vi "control final.vi"() -> ()   [LabVIEW 2013]
uses:
  <vilib>/userdefined/High Color/IMAQdx.ctl
  <vilib>/LabVIEW Interface for Arduino/Type Defs/Board Type.ctl
  <vilib>/LabVIEW Interface for Arduino/Type Defs/Connection Type.ctl
  <vilib>/LabVIEW Interface for Arduino/Type Defs/Pin Mode.ctl
  <vilib>/Utility/inputDevices.llb/closeJoystick.vi
  <vilib>/Utility/inputDevices.llb/joystickAcquire.vi
  <vilib>/LabVIEW Interface for Arduino/LabVIEW Interface for Arduino.lvlib
  <vilib>/vision/driver/NI_Vision_Acquisition_Software.lvlib
panel:
  in  "light  2":bool
  in  "light  2":bool
  in  "Session In":T1
  in  "?":bool
  out "CAMERA":T2(plugin-control)
  in  "throtel":dbl(knob) scale=0.0..180.0
  in  "cacamera 2":dbl(knob) scale=0.0..180.0
  in  "laser":bool
  in  "P":bool
  in  "light":bool
  in  "M":bool
  in  "PWM":dbl(knob) scale=0.0..180.0
  out "Voltage":dbl(knob) scale=0.0..5.0
  out "throtel":dbl(knob) scale=0.0..180.0
  out "camera":dbl(knob) scale=0.0..180.0
  out "up":bool
  out "dwn":bool
  out "Rot right":bool
  out "Rot left":bool
  out "gripper":dbl(knob) scale=0.0..180.0
  in  "gripper":dbl(knob) scale=0.0..180.0
  in  "VISA resource":refnum<visa-resource-name>
  out "left":bool
  out "backword":bool
  out "right":bool
  out "forward":bool
  in  "stop":bool
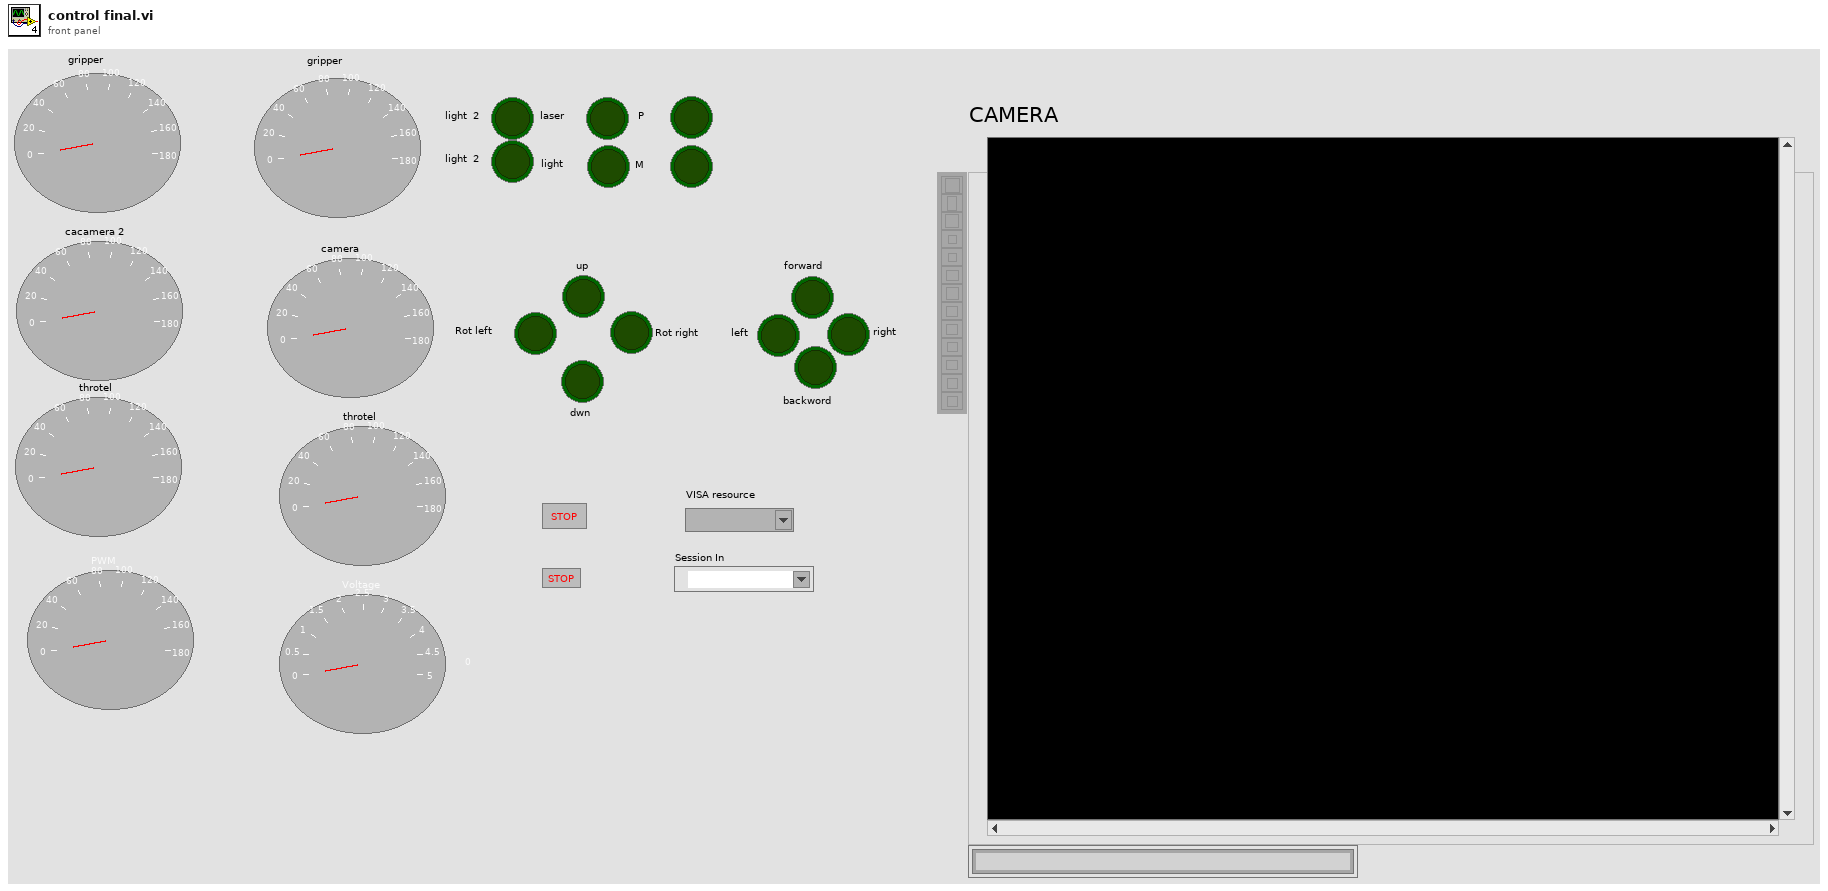
[diagram p1: front panel]
types:
  T1 = typedef "IMAQdx.ctl" = refnum<k21>
  T2 = typedef "IMAQ Image.ctl" = refnum<image>
  T3 = typedef "Image Type" = u32
  T4 = typedef "LabVIEW Interface for Arduino.lvlib/Pin Mode.ctl" = enum8{"Input", "Output"}
  T5 = typedef "LabVIEW Interface for Arduino.lvlib/Connection Type.ctl" = enum8{"USB / Serial", "XBEE", "BlueSmirf (Bluetooth)"}
  T6 = typedef "LabVIEW Interface for Arduino.lvlib/Board Type.ctl" = enum16{"Uno", "Dimuelanove w/Atmega 328", "Mega 2560"}
  T7 = typedef "LabVIEW Interface for Arduino.lvlib/Arduino Resource.ctl" = cluster{"VISA resource":refnum<visa-resource-name>, "Board Type":T6, "Connection Type":enum8{"USB / Serial"}, "Bytes Per Packet (15)":u8}
  T8 = cluster{"X axis":i32, "Y axis":i32, "Z axis":i32, "X axis rotation":i32, "Y axis rotation":i32, "Z axis rotation":i32, "U axis":i32, "V axis":i32}
  T9 = cluster{"button 1":bool, "button 2":bool, "button 3":bool, "button 4":bool, "button 5":bool, "button 6":bool, "button 7":bool, "button 8":bool, "button 9":bool, "button 10":bool, "button 11":bool, "button 12":bool, "button 13":bool, "button 14":bool, "button 15":bool, "button 16":bool, "button 17":bool, "button 18":bool, "button 19":bool, "button 20":bool, "button 21":bool, "button 22":bool, "button 23":bool, "button 24":bool, "button 25":bool, "button 26":bool, "button 27":bool, "button 28":bool, "button 29":bool, "button 30":bool, "button 31":bool, "button 32":bool}
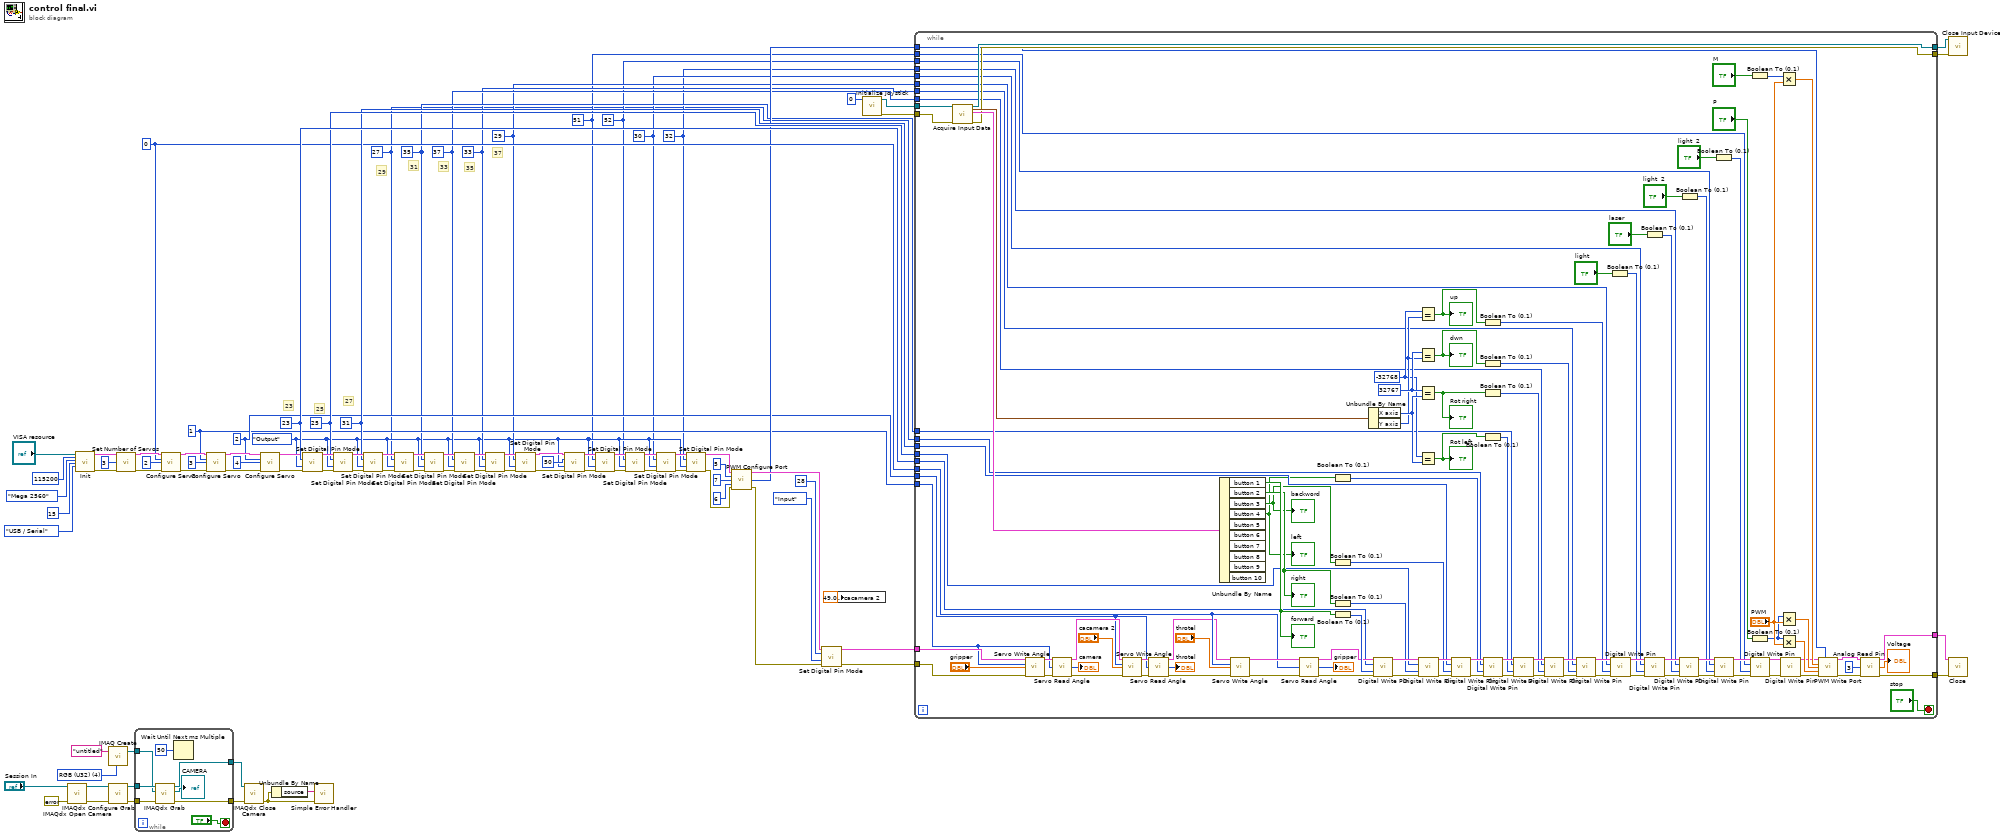
[diagram p0: block diagram]
diagram:
  w8 = T3 4 items=["Grayscale (U8)", "Grayscale (I16)", "Grayscale (SGL)", "Complex (CSG)", "RGB (U32)", "HSL (U32)", "RGB (U64)", "Grayscale (U16)"] ("Image Type")
  w19 = u8 30 ("Digital I/O Pin")
  w18 = u8 32 ("Digital I/O Pin")
  w4 = u8 52 ("Digital I/O Pin")
  w3 = u8 51 ("Digital I/O Pin")
  w24 = u8 29 ("Digital I/O Pin")
  w25 = u8 33 ("Digital I/O Pin")
  w26 = u8 37 ("Digital I/O Pin")
  w27 = u8 35 ("Digital I/O Pin")
  w30 = u8 2 ("Servo Number (0)")
  w29 = u8 1 ("Servo Number (0)")
  w2 = u8 27 ("Value (0)")
  w68 = u8 31 ("Value (0)")
  w69 = u8 25 ("Value (0)")
  w70 = u8 23 ("Value (0)")
  w20 = Pin_Mode."Output" ("Pin Mode (Input)")
  w67 = u8 0 ("Servo Number")
  # "23"
  # "25"
  # "37"
  # "35"
  # "33"
  # "31"
  # "29"
  # "27"
  n1 = call <vilib>:"IMAQdx Open Camera.vi"("error in"=errorcluster {"status"=FALSE, "code"=0, "source"=""}, "Session In"="Session In") -> ("error out"=w12:errorcluster, "Session Out"=w13:T1)  [unwired: 8 in]
  n2 = call <vilib>:"Init.vi"("VISA resource"="VISA resource", "Baud Rate (115200)"=u32 115200, "Board Type (Uno)"=Board_Type."Mega 2560", "Bytes Per Packet (15)"=u32 15, "Connection Type (USB/Serial)"=Connection_Type."USB / Serial") -> ("Arduino Resource"=w78:T7, "error out"=w77:errorcluster)  [unwired: 13 in]
  n3 = call "IMAQ Create"("Image Name"="untitled", "Image Type"=w8) -> ("New Image"=w7:T2)  [unwired: 3 in, 1 out]
  n4 = call <vilib>:"IMAQdx Configure Grab.vi"("error in"=w12, "Session In"=w13) -> ("error out"=w11:errorcluster, "Session Out"=w10:T1)  [unwired: 8 in]
  n5 = call <vilib>:"Set Number of Servos.vi"("Arduino Resource"=w78, "Number Of Servos (1)"=u8 3, "error in"=w77) -> ("Arduino Resource"=w82:T7, "error out"=w81:errorcluster)  [unwired: 11 in]
  n6 = while {
    tunnel: w10 -> [w100]
    tunnel: w11 -> [w99]
    tunnel: [w98] -> w15
    tunnel: [w97] -> w14
    tunnel: w7 -> [w96]
    stop <- "?" stop-if-true
    n7 = call <vilib>:"IMAQdx Grab.vi"("error in"=w99, "Image In"=w96, "Session In"=w100) -> ("error out"=w98:errorcluster, "Image Out"=→"CAMERA":T2, "Session Out"=w97:T1)  [unwired: 5 in, 1 out]
    n8 = Wait Until Next ms Multiple(millisecond multiple=u32 50) -> ()  [unwired: 1 out]
  }
  n9 = call <vilib>:"Configure Servo.vi"("Arduino Resource"=w82, "Servo Number (0)"=w67, "DIO Pin (2)"=u8 2 ("Servo Number"), "error in"=w81) -> ("Arduino Resource"=w51:T7, "error out"=w47:errorcluster)  [unwired: 10 in]
  n10 = call <vilib>:"Configure Servo.vi"("Arduino Resource"=w51, "Servo Number (0)"=w29, "DIO Pin (2)"=u8 3, "error in"=w47) -> ("Arduino Resource"=w50:T7, "error out"=w46:errorcluster)  [unwired: 10 in]
  n11 = call <vilib>:"IMAQdx Close Camera.vi"("error in"=w15, "Session In"=w14) -> ("error out"=w6:errorcluster)  [unwired: 9 in]
  n12 = call <vilib>:"Configure Servo.vi"("Arduino Resource"=w50, "Servo Number (0)"=w30, "DIO Pin (2)"=u8 4, "error in"=w46) -> ("Arduino Resource"=w49:T7, "error out"=w48:errorcluster)  [unwired: 10 in]
  n13 = Unbundle By Name(w6) -> ("source"=w5:string)
  n14 = call <vilib>:"Set Digital Pin Mode.vi"("Arduino Resource"=w49, "Digital I/O Pin"=w70, "Pin Mode (Input)"=w20, "error in"=w48) -> ("Arduino Resource"=w76:T7, "error out"=w71:errorcluster)  [unwired: 10 in]
  n15 = call <vilib>:"Simple Error Handler.vi"("error source (\" \")"=w5, "error in (no error)"=w6) -> ()  [unwired: 3 in, 5 out]
  n16 = call <vilib>:"Set Digital Pin Mode.vi"("Arduino Resource"=w76, "Digital I/O Pin"=w69, "Pin Mode (Input)"=w20, "error in"=w71) -> ("Arduino Resource"=w75:T7, "error out"=w72:errorcluster)  [unwired: 10 in]
  n17 = call <vilib>:"Set Digital Pin Mode.vi"("Arduino Resource"=w75, "Digital I/O Pin"=w68, "Pin Mode (Input)"=w20, "error in"=w72) -> ("Arduino Resource"=w74:T7, "error out"=w73:errorcluster)  [unwired: 10 in]
  n18 = call <vilib>:"Set Digital Pin Mode.vi"("Arduino Resource"=w74, "Digital I/O Pin"=w2, "Pin Mode (Input)"=w20, "error in"=w73) -> ("Arduino Resource"=w65:T7, "error out"=w52:errorcluster)  [unwired: 10 in]
  n19 = call <vilib>:"Set Digital Pin Mode.vi"("Arduino Resource"=w65, "Digital I/O Pin"=w27, "Pin Mode (Input)"=w20, "error in"=w52) -> ("Arduino Resource"=w64:T7, "error out"=w53:errorcluster)  [unwired: 10 in]
  n20 = call <vilib>:"Set Digital Pin Mode.vi"("Arduino Resource"=w64, "Digital I/O Pin"=w26, "Pin Mode (Input)"=w20, "error in"=w53) -> ("Arduino Resource"=w63:T7, "error out"=w54:errorcluster)  [unwired: 10 in]
  n21 = call <vilib>:"Set Digital Pin Mode.vi"("Arduino Resource"=w63, "Digital I/O Pin"=w25, "Pin Mode (Input)"=w20, "error in"=w54) -> ("Arduino Resource"=w62:T7, "error out"=w55:errorcluster)  [unwired: 10 in]
  n22 = call <vilib>:"Set Digital Pin Mode.vi"("Arduino Resource"=w62, "Digital I/O Pin"=w24, "Pin Mode (Input)"=w20, "error in"=w55) -> ("Arduino Resource"=w61:T7, "error out"=w56:errorcluster)  [unwired: 10 in]
  n23 = call <vilib>:"Set Digital Pin Mode.vi"("Arduino Resource"=w61, "Digital I/O Pin"=u8 50, "Pin Mode (Input)"=w20, "error in"=w56) -> ("Arduino Resource"=w60:T7, "error out"=w57:errorcluster)  [unwired: 10 in]
  n24 = call <vilib>:"Set Digital Pin Mode.vi"("Arduino Resource"=w60, "Digital I/O Pin"=w3, "Pin Mode (Input)"=w20, "error in"=w57) -> ("Arduino Resource"=w59:T7, "error out"=w58:errorcluster)  [unwired: 10 in]
  n25 = call <vilib>:"Set Digital Pin Mode.vi"("Arduino Resource"=w59, "Digital I/O Pin"=w4, "Pin Mode (Input)"=w20, "error in"=w58) -> ("Arduino Resource"=w22:T7, "error out"=w21:errorcluster)  [unwired: 10 in]
  n26 = call <vilib>:"Set Digital Pin Mode.vi"("Arduino Resource"=w22, "Digital I/O Pin"=w19, "Pin Mode (Input)"=w20, "error in"=w21) -> ("Arduino Resource"=w40:T7, "error out"=w39:errorcluster)  [unwired: 10 in]
  n27 = call <vilib>:"Set Digital Pin Mode.vi"("Arduino Resource"=w40, "Digital I/O Pin"=w18, "Pin Mode (Input)"=w20, "error in"=w39) -> ("Arduino Resource"=w38:T7, "error out"=w37:errorcluster)  [unwired: 10 in]
  n28 = call <vilib>:"PWM Configure Port.vi"("Arduino Resource"=w38, "PWM Pin (3)"=u8 5, "PWM Pin (5)"=u8 7, "PWM Pin (6)"=u8 6, "error in"=w37) -> ("Arduino Resource"=w35:T7, "PWM Pins"=w31:u8[], "error out"=w36:errorcluster)  [unwired: 8 in]
  n29 = call <vilib>:"Set Digital Pin Mode.vi"("Arduino Resource"=w35, "Digital I/O Pin"=u8 28, "Pin Mode (Input)"=Pin_Mode."Input", "error in"=w36) -> ("Arduino Resource"=w42:T7, "error out"=w43:errorcluster)  [unwired: 10 in]
  n30 = local write "cacamera 2"(49.0 ("caca 2")) -> ()
  n31 = call <vilib>:"Initialize Joystick.vi"("device index"=0) -> ("error out"=w88:errorcluster, "device ID"=w89:refnum<k1>)  [unwired: 9 in]
  n32 = while {
    tunnel: w89 -> [w211]
    tunnel: w88 -> [w210]
    tunnel: [w167] -> w87
    tunnel: [w166] -> w86
    tunnel: [w203] -> w85
    tunnel: [w202] -> w84
    tunnel: w70 -> [w175]
    tunnel: w69 -> [w174]
    tunnel: w68 -> [w173]
    tunnel: w2 -> [w172]
    tunnel: w67 -> [w171]
    tunnel: w42 -> [w144]
    tunnel: w43 -> [w143]
    tunnel: w31 -> [w154]
    tunnel: w30 -> [w139]
    tunnel: w29 -> [w140]
    tunnel: w27 -> [w138]
    tunnel: w26 -> [w137]
    tunnel: w25 -> [w136]
    tunnel: w24 -> [w135]
    tunnel: w19 -> [w120]
    tunnel: w18 -> [w119]
    tunnel: w4 -> [w104]
    tunnel: w3 -> [w103]
    stop <- "stop" stop-if-true
    w204 = -32768 ("x")
    w206 = 32767 ("x")
    n33 = call-poly <vilib>:"Acquire Input Data.vi"("device ID"=w211, "error in (no error)"=w210) -> ("device ID"=w203:refnum<k1>, "axis info"=w208:T8, "button info"=w209:T9, "error out"=w202:errorcluster)  [unwired: 13 in, 1 out]
    n34 = call <vilib>:"Servo Write Angle.vi"("Arduino Resource"=w144, "Servo Number"=w140, "Angle (Degrees)"="gripper", "error in"=w143) -> ("Arduino Resource"=w149:T7, "error out"=w152:errorcluster)  [unwired: 10 in]
    n35 = call <vilib>:"Servo Read Angle.vi"("Arduino Resource"=w149, "Servo Number"=w140, "error in"=w152) -> ("Arduino Resource"=w150:T7, "Angle (Degrees)"=→"camera":u8, "error out"=w148:errorcluster)  [unwired: 10 in]
    n36 = call <vilib>:"Servo Write Angle.vi"("Arduino Resource"=w150, "Servo Number"=w139, "Angle (Degrees)"="cacamera 2", "error in"=w148) -> ("Arduino Resource"=w151:T7, "error out"=w153:errorcluster)  [unwired: 10 in]
    n37 = call <vilib>:"Servo Read Angle.vi"("Arduino Resource"=w151, "Servo Number"=w139, "error in"=w153) -> ("Arduino Resource"=w146:T7, "Angle (Degrees)"=→"throtel":u8, "error out"=w147:errorcluster)  [unwired: 10 in]
    n38 = Unbundle By Name(w209) -> ("button 1"=w201:bool, "button 2"=w200:bool, "button 3"=w199:bool, "button 4"=w129:bool)  [unwired: 6 out]
    "forward" <- w201
    "right" <- w200
    "backword" <- w199
    "left" <- w129
    n39 = call <vilib>:"Servo Write Angle.vi"("Arduino Resource"=w146, "Servo Number"=w171, "Angle (Degrees)"="throtel", "error in"=w147) -> ("Arduino Resource"=w179:T7, "error out"=w178:errorcluster)  [unwired: 10 in]
    n40 = call <vilib>:"Servo Read Angle.vi"("Arduino Resource"=w179, "Servo Number"=w171, "error in"=w178) -> ("Arduino Resource"=w177:T7, "Angle (Degrees)"=→"gripper":u8, "error out"=w176:errorcluster)  [unwired: 10 in]
    n41 = Boolean To (0,1)(Boolean=w129) -> (0, 1=w184:i16)
    n42 = Boolean To (0,1)(Boolean=w199) -> (0, 1=w183:i16)
    n43 = Boolean To (0,1)(Boolean=w200) -> (0, 1=w182:i16)
    n44 = Boolean To (0,1)(Boolean=w201) -> (0, 1=w181:i16)
    n45 = Unbundle By Name(w208) -> ("X axis"=w207:i32, "Y axis"=w205:i32)
    n46 = call <vilib>:"Digital Write Pin.vi"("Arduino Resource"=w177, "Digital I/O Pin (0)"=w175, "Value (0)"=w181, "error in"=w176) -> ("Arduino Resource"=w193:T7, "error out"=w196:errorcluster)  [unwired: 10 in]
    n47 = Equal?(x=w204, y=w205) -> (x = y?=w160:bool)
    "up" <- w160
    n48 = Equal?(x=w206, y=w205) -> (x = y?=w161:bool)
    "dwn" <- w161
    n49 = Equal?(x=w206, y=w207) -> (x = y?=w162:bool)
    "Rot right" <- w162
    n50 = Equal?(x=w204, y=w207) -> (x = y?=w163:bool)
    "Rot left" <- w163
    n51 = call <vilib>:"Digital Write Pin.vi"("Arduino Resource"=w193, "Digital I/O Pin (0)"=w174, "Value (0)"=w182, "error in"=w196) -> ("Arduino Resource"=w198:T7, "error out"=w195:errorcluster)  [unwired: 10 in]
    n52 = call <vilib>:"Digital Write Pin.vi"("Arduino Resource"=w198, "Digital I/O Pin (0)"=w173, "Value (0)"=w183, "error in"=w195) -> ("Arduino Resource"=w197:T7, "error out"=w194:errorcluster)  [unwired: 10 in]
    n53 = Boolean To (0,1)(Boolean=w160) -> (0, 1=w102:i16)
    n54 = Boolean To (0,1)(Boolean=w161) -> (0, 1=w157:i16)
    n55 = Boolean To (0,1)(Boolean=w162) -> (0, 1=w158:i16)
    n56 = Boolean To (0,1)(Boolean=w163) -> (0, 1=w159:i16)
    n57 = call <vilib>:"Digital Write Pin.vi"("Arduino Resource"=w197, "Digital I/O Pin (0)"=w172, "Value (0)"=w184, "error in"=w194) -> ("Arduino Resource"=w169:T7, "error out"=w168:errorcluster)  [unwired: 10 in]
    n58 = call <vilib>:"Digital Write Pin.vi"("Arduino Resource"=w169, "Digital I/O Pin (0)"=w138, "Value (0)"=w159, "error in"=w168) -> ("Arduino Resource"=w185:T7, "error out"=w189:errorcluster)  [unwired: 10 in]
    n59 = call <vilib>:"Digital Write Pin.vi"("Arduino Resource"=w185, "Digital I/O Pin (0)"=w137, "Value (0)"=w158, "error in"=w189) -> ("Arduino Resource"=w192:T7, "error out"=w188:errorcluster)  [unwired: 10 in]
    n60 = call <vilib>:"Digital Write Pin.vi"("Arduino Resource"=w192, "Digital I/O Pin (0)"=w136, "Value (0)"=w157, "error in"=w188) -> ("Arduino Resource"=w191:T7, "error out"=w187:errorcluster)  [unwired: 10 in]
    n61 = Boolean To (0,1)(Boolean="light") -> (0, 1=w122:i16)
    n62 = call <vilib>:"Digital Write Pin.vi"("Arduino Resource"=w191, "Digital I/O Pin (0)"=w135, "Value (0)"=w102, "error in"=w187) -> ("Arduino Resource"=w190:T7, "error out"=w186:errorcluster)  [unwired: 10 in]
    n63 = Boolean To (0,1)(Boolean="laser") -> (0, 1=w121:i16)
    n64 = call <vilib>:"Digital Write Pin.vi"("Arduino Resource"=w190, "Digital I/O Pin (0)"=w120, "Value (0)"=w122, "error in"=w186) -> ("Arduino Resource"=w165:T7, "error out"=w164:errorcluster)  [unwired: 10 in]
    n65 = Boolean To (0,1)(Boolean="light  2") -> (0, 1=w105:i16)
    n66 = call <vilib>:"Digital Write Pin.vi"("Arduino Resource"=w165, "Digital I/O Pin (0)"=w119, "Value (0)"=w121, "error in"=w164) -> ("Arduino Resource"=w110:T7, "error out"=w109:errorcluster)  [unwired: 10 in]
    n67 = Boolean To (0,1)(Boolean="light  2") -> (0, 1=w106:i16)
    n68 = call <vilib>:"Digital Write Pin.vi"("Arduino Resource"=w110, "Digital I/O Pin (0)"=w104, "Value (0)"=w105, "error in"=w109) -> ("Arduino Resource"=w112:T7, "error out"=w111:errorcluster)  [unwired: 10 in]
    n69 = Boolean To (0,1)(Boolean="M") -> (0, 1=w125:i16)
    n70 = Boolean To (0,1)(Boolean="P") -> (0, 1=w126:i16)
    n71 = call <vilib>:"Digital Write Pin.vi"("Arduino Resource"=w112, "Digital I/O Pin (0)"=w103, "Value (0)"=w106, "error in"=w111) -> ("Arduino Resource"=w114:T7, "error out"=w113:errorcluster)  [unwired: 10 in]
    n72 = Multiply(x=w125, y="PWM") -> (x*y=w132:dbl)
    n73 = Multiply(x=w126, y="PWM") -> (x*y=w131:dbl)
    n74 = Multiply(x=w126, y="PWM") -> (x*y=w130:dbl)
    n75 = call <vilib>:"Digital Write Pin.vi"("Arduino Resource"=w114, "error in"=w113) -> ("Arduino Resource"=w116:T7, "error out"=w115:errorcluster)  [unwired: 12 in]
    n76 = call <vilib>:"PWM Write Port.vi"("Arduino Resource"=w116, "PWM Pins"=w154, "PWM 0 (0-255)"=w132, "PWM 1 (0-255)"=w131, "PWM 2 (0-255)"=w130, "error in"=w115) -> ("Arduino Resource"=w156:T7, "error out"=w155:errorcluster)  [unwired: 7 in, 1 out]
    n77 = call <vilib>:"Analog Read Pin.vi"("Arduino Resource"=w156, "Analog Input Pin (0)"=u8 3, "error in"=w155) -> ("Arduino Resource"=w167:T7, "Voltage"=→"Voltage":dbl, "error out"=w166:errorcluster)  [unwired: 10 in]
  }
  n78 = call-poly <vilib>:"Close Input Device.vi"("error in (no error)"=w84, "device ID"=w85) -> ()  [unwired: 8 in, 1 out]
  n79 = call <vilib>:"Close.vi"("Arduino Resource"=w87, "error in"=w86) -> ()  [unwired: 13 in, 1 out]
